vi "monochromatorCommandGetGratingLines.vi"(8 "error in":errorcluster, 10 "grating":i32, 11 "monochromator":refnum<k24>) -> (0 "error out":errorcluster, 2 "grating_lines":i32, 3 "monochromator":refnum<k24>)   [LabVIEW 2009]
doc: "Get Grating Lines"
uses:
  C:/Users/anderson.chen/Desktop/Software Development/Cornerstone Series API (LV9)/Cornerstone DLL/Cornerstone.dll
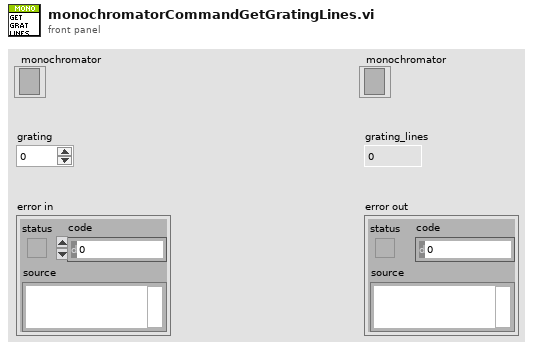
[diagram p1: front panel]
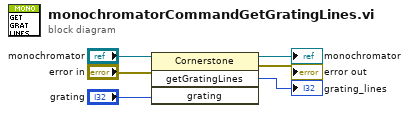
[diagram p0: block diagram]
diagram:
  n1 = invoke class="Cornerstone" method="getGratingLines"(reference="monochromator", error in="error in", "grating"="grating") -> (reference out=→"monochromator":refnum<k24>, error out=→"error out":errorcluster, "getGratingLines"=→"grating_lines":i32)  [unwired: 1 in, 1 out]
